vi "Set Personality.vi"(0 "GEA2 Reference In":refnum<k24>, 1 "Expected Version":string, 5 "Expected Personality":u8, 7 "Expected Model ID":u8, 11 "Error In":errorcluster) -> (3 "Actual Personality":u8, 4 "GEA2 Reference Out":refnum<k24>, 6 "Pass/Fail?":bool=TRUE, 8 "Report Text":string, 10 "Actual Version":string, 14 "Actual Model ID":u8, 15 "Error Out":errorcluster)   [LabVIEW 2016]
doc: "Use this VI to set the washer personality."
uses:
  C:/Automation/DLLs/PC Dot Net/GeaCommunication.dll
  Common/LabVIEW GEA2 Toolkit/LabVIEW_GEA2_Toolkit.lvlibp/type defs/Source_Destination.ctl
  Common/LabVIEW GEA2 Toolkit/LabVIEW_GEA2_Toolkit.lvlibp/type defs/ERD Read Data In.ctl
  Common/LabVIEW GEA2 Toolkit/LabVIEW_GEA2_Toolkit.lvlibp/type defs/Data Type.ctl
  Common/LabVIEW GEA2 Toolkit/LabVIEW_GEA2_Toolkit.lvlibp/type defs/ERD Write Data In.ctl
  Common/LabVIEW GEA2 Toolkit/LabVIEW_GEA2_Toolkit.lvlibp
  Automation/Product Specific/Clothes Care/TL27/Projects/TL27.lvlib
panel:
  in  "Standalone?":bool
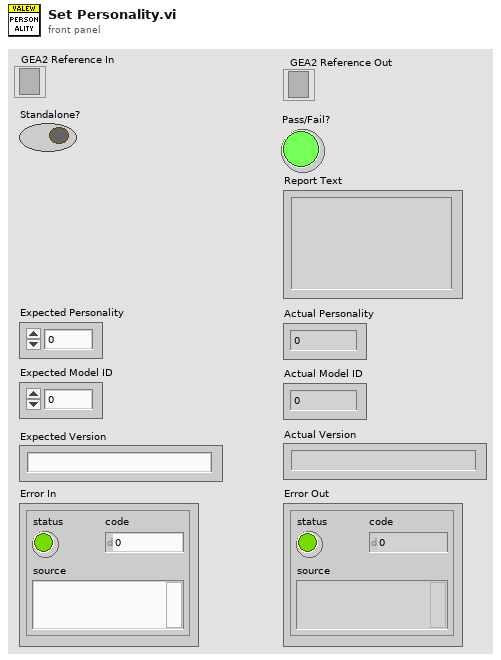
[diagram p1: front panel]
types:
  T1 = typedef "LabVIEW_GEA2_Toolkit.lvlibp/ERD Read Data In.ctl" = cluster{"ERD Number":u16, "Data Type":T2}
  T2 = typedef "LabVIEW_GEA2_Toolkit.lvlibp/Data Type.ctl" = enum16{"string", "boolean", "uint8_t", "uint16_t", "uint32_t", "uint64_t", "int8_t", "int16_t", "int32_t", "int64_t"}
  T3 = typedef "LabVIEW_GEA2_Toolkit.lvlibp/Source_Destination.ctl" = cluster{"Source":u8, "Destination":u8}
  T4 = typedef "LabVIEW_GEA2_Toolkit.lvlibp/ERD Read Data Out.ctl" = cluster{"ERD Number":u16, "Data":string}
  T5 = typedef "LabVIEW_GEA2_Toolkit.lvlibp/ERD Write Data In.ctl" = cluster{"ERD Number":u16, "Data Type":T2, "Data":string}
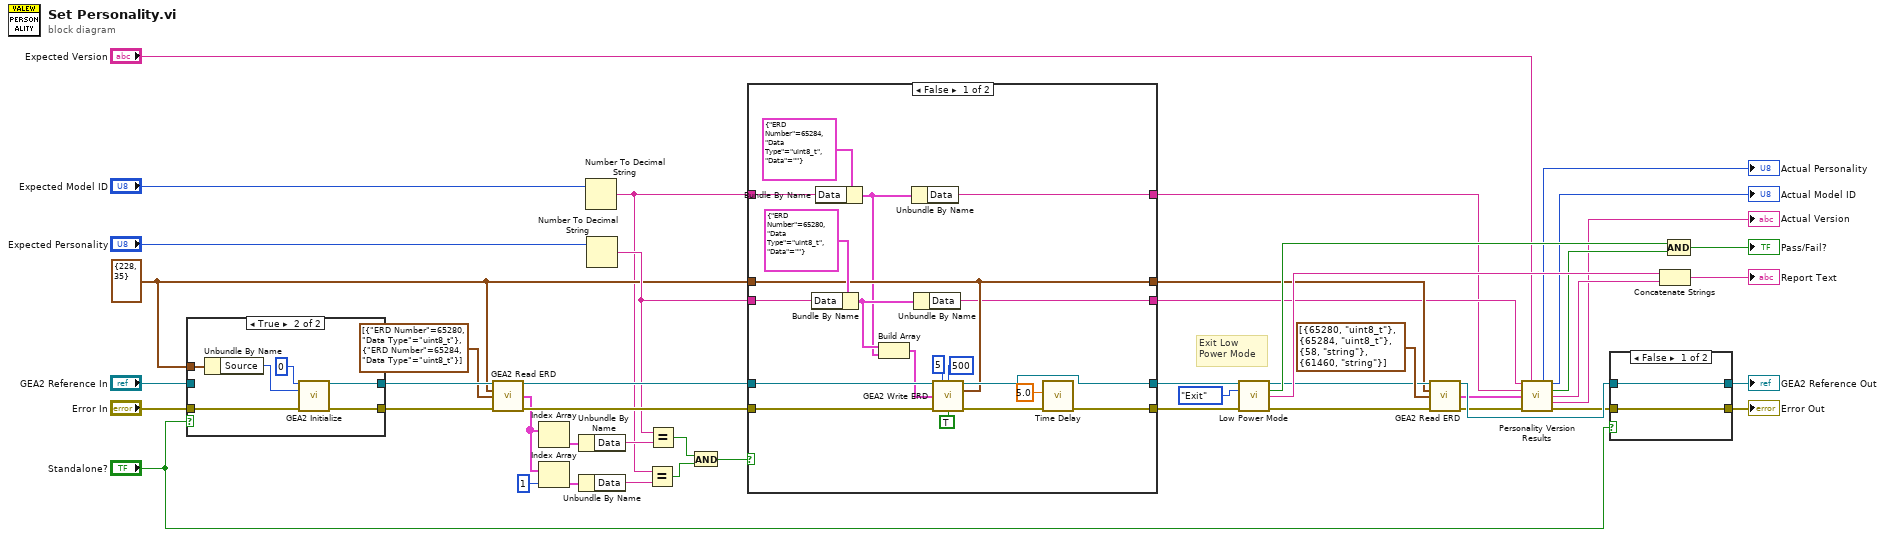
[diagram p0: block diagram]
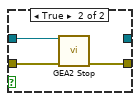
[diagram p3: hidden frame]
diagram:
  w26 = T3 {"Source"=228, "Destination"=35} ("GEA Inputs")
  # "Exit Low \nPower Mode"
  n1 = case shown="True" "Standalone?" {
    tunnel: "Error In" -> [w48 w55]
    tunnel: [w48 w54] -> w33
    tunnel: "GEA2 Reference In" -> [w49 _]
    tunnel: [w49 w53] -> w34
    tunnel: w26 -> [_ w51]
    frame False {
    }
    frame True {
      n2 = Unbundle By Name(w51) -> ("Source"=w52:u8)
      n3 = call "GEA2 Initialize.vi"("Board Index"=0, "Source Address"=w52, "error in"=w55) -> ("GEA2 Reference Out"=w53:refnum<k24>, "error out"=w54:errorcluster)  [unwired: 10 in, 1 out]
    }
  }
  n4 = call "GEA2 Read ERD.vi"("GEA2 Reference In"=w34, "GEA Inputs"=w26, "Read ERD List"=T1[] [{"ERD Number"=65280, "Data Type"=enum."uint8_t"}, {"ERD Number"=65284, "Data Type"=enum."uint8_t"}], "Error In"=w33) -> ("GEA2 Reference Out"=w32:refnum<k24>, "ERD Data Out"=w15:T4[], "Error Out"=w31:errorcluster)  [unwired: 8 in, 1 out]
  n5 = Index Array(array=w15) -> (element=w30:T4)  [unwired: 1 in]
  n6 = Index Array(array=w15, index=1) -> (element=w14:T4)
  n7 = Unbundle By Name(w30) -> ("Data"=w28:string)
  n8 = Unbundle By Name(w14) -> ("Data"=w13:string)
  n9 = Number To Decimal String(number="Expected Model ID") -> (decimal integer string=w12:string)  [unwired: 1 in]
  n10 = Number To Decimal String(number="Expected Personality") -> (decimal integer string=w27:string)  [unwired: 1 in]
  n11 = Equal?(x=w12, y=w13) -> (x = y?=w19:bool)
  n12 = Equal?(x=w27, y=w28) -> (x = y?=w18:bool)
  n13 = And(x=w18, y=w19) -> (x .and. y?=w17:bool)
  n14 = case shown="False" w17 {
    tunnel: [w57 w78] -> w42
    tunnel: [w74 w79] -> w39
    tunnel: w32 -> [w73 w79]
    tunnel: w31 -> [w72 w78]
    tunnel: w27 -> [w69 w76]
    tunnel: w26 -> [w68 w77]
    tunnel: [w68 w77] -> w21
    tunnel: [w66 w76] -> w9
    tunnel: w12 -> [w62 w75]
    tunnel: [w56 w75] -> w8
    frame False {
      n15 = Bundle By Name(cluster=T5 {"ERD Number"=65280, "Data Type"=enum."uint8_t", "Data"=""} ("ERD Write Data In"), "Data"=w69) -> (w67:T5)
      n16 = Bundle By Name(cluster=T5 {"ERD Number"=65284, "Data Type"=enum."uint8_t", "Data"=""} ("ERD Write Data In"), "Data"=w62) -> (w60:T5)
      n17 = Build Array(w67, w60) -> (w70:T5[])
      n18 = Unbundle By Name(w60) -> ("Data"=w56:string)
      n19 = Unbundle By Name(w67) -> ("Data"=w66:string)
      n20 = call "GEA2 Write ERD.vi"("GEA2 Reference In"=w73, "# of Tries"=5 ("Retry Count"), "Read Timeout (ms)"=u32 500, "GEA Inputs"=w68, "Write ERD List"=w70, "Error In"=w72, "Verify ERD Response?"=TRUE) -> ("GEA2 Reference Out"=w74:refnum<k24>, "Error Out"=w58:errorcluster)  [unwired: 6 in, 1 out]
      n21 = call "Time Delay"("error in (no error)"=w58, "Delay Time (s)"=5.0) -> ("error out"=w57:errorcluster)  [unwired: 9 in]
    }
    frame True {
    }
  }
  n22 = call "Low Power Mode.vi"("GEA2 Reference In"=w39, "Action"=enum16{"Enter", "Exit"}."Exit", "Error In"=w42) -> ("GEA2 Reference Out"=w24:refnum<k24>, "Pass/Fail?"=w37:bool, "Report Text"=w41:string, "Error Out"=w23:errorcluster)  [unwired: 9 in]
  n23 = call "GEA2 Read ERD.vi"("GEA2 Reference In"=w24, "GEA Inputs"=w21, "Read ERD List"=T1[] [{"ERD Number"=65280, "Data Type"=enum."uint8_t"}, {"ERD Number"=65284, "Data Type"=enum."uint8_t"}, {"ERD Number"=58, "Data Type"=enum."string"}, {"ERD Number"=61460, "Data Type"=enum."string"}], "Error In"=w23) -> ("GEA2 Reference Out"=w22:refnum<k24>, "ERD Data Out"=w6:T4[], "Error Out"=w11:errorcluster)  [unwired: 8 in, 1 out]
  n24 = call "Personality Version Results.vi"("Expected Personality"=w9, "Expected Version"="Expected Version", "Expected Model"=w8, "ERD Data Out"=w6, "Error In"=w11) -> ("Actual Personality"=→"Actual Personality":u8, "Actual Model ID"=→"Actual Model ID":u8, "Boolean"=w5:bool, "Report Text"=w4:string, "Actual Version"=→"Actual Version":string, "Error Out"=w10:errorcluster)  [unwired: 5 in]
  n25 = case shown="False" "Standalone?" {
    tunnel: [w80 w84] -> w47
    tunnel: [w81 _] -> w46
    tunnel: w22 -> [w81 w83]
    tunnel: w10 -> [w80 w82]
    frame False {
    }
    frame True {
      n26 = call "GEA2 Stop.vi"("GEA2 Reference In"=w83, "Error In"=w82) -> ("Error Out"=w84:errorcluster)  [unwired: 13 in]
    }
  }
  "Error Out" <- w47
  "GEA2 Reference Out" <- w46
  n27 = Concatenate Strings(w41, w4) -> (→"Report Text":string)
  n28 = Compound Arithmetic op=AND(w37, w5) -> (→"Pass/Fail?":bool)
